vi "GetSelectedRelayCycles.vi"(2 "error in (no error)":errorcluster) -> (0 "error out":errorcluster, 1 "StringOfRelayCycles":string)   [LabVIEW 2009]
doc: "Produce a string containing about 15 cycle counts from selected relays"
panel:
  out "AT3_10dB7141RelayCycles 2":i32
  out "S2ToTransferSw5141RelayCycles":i32
  out "S1ToTransferSw5166RelayCycles":i32
  out "TxDetector1038RelayCycles":i32
  out "TxDisable7221RelayCycles":i32
  out "WGOutToAnt7206RelayCycles":i32
  out "Pwr15Supply1039RelayCycles":i32
  out "BoxInTemp1019RelayCycles":i32
  out "TransferSw7121RelayCycles":i32
  out "AT5_2dBSteps7161RelayCycles":i32
  out "AT4_10dBSteps7165RelayCycles":i32
  out "AmpBypass7201RelayCycles":i32
  out "S3toSpllitter5123RelayCycles":i32
  out "S5toPwrSensor7103RelayCycles":i32
  out "S4toSigGen5102RelayCycles":i32
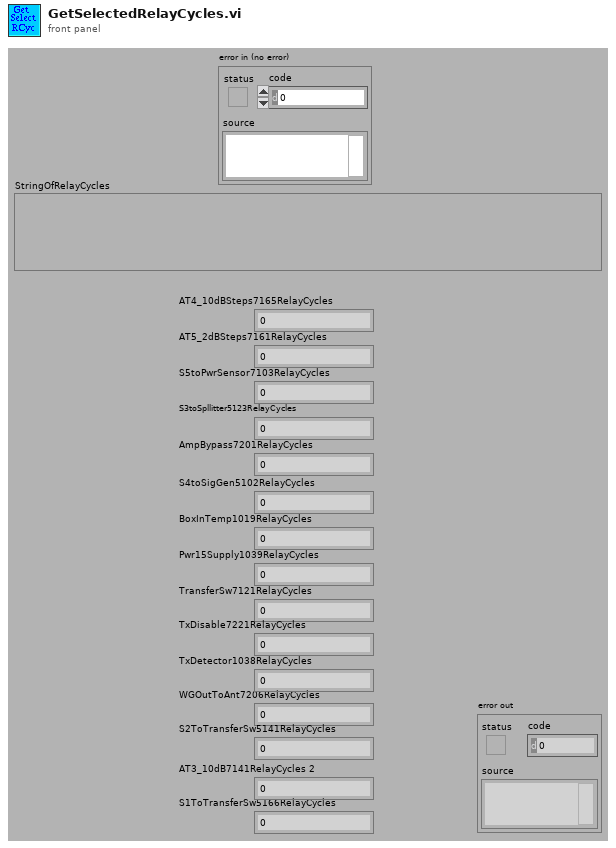
[diagram p1: front panel]
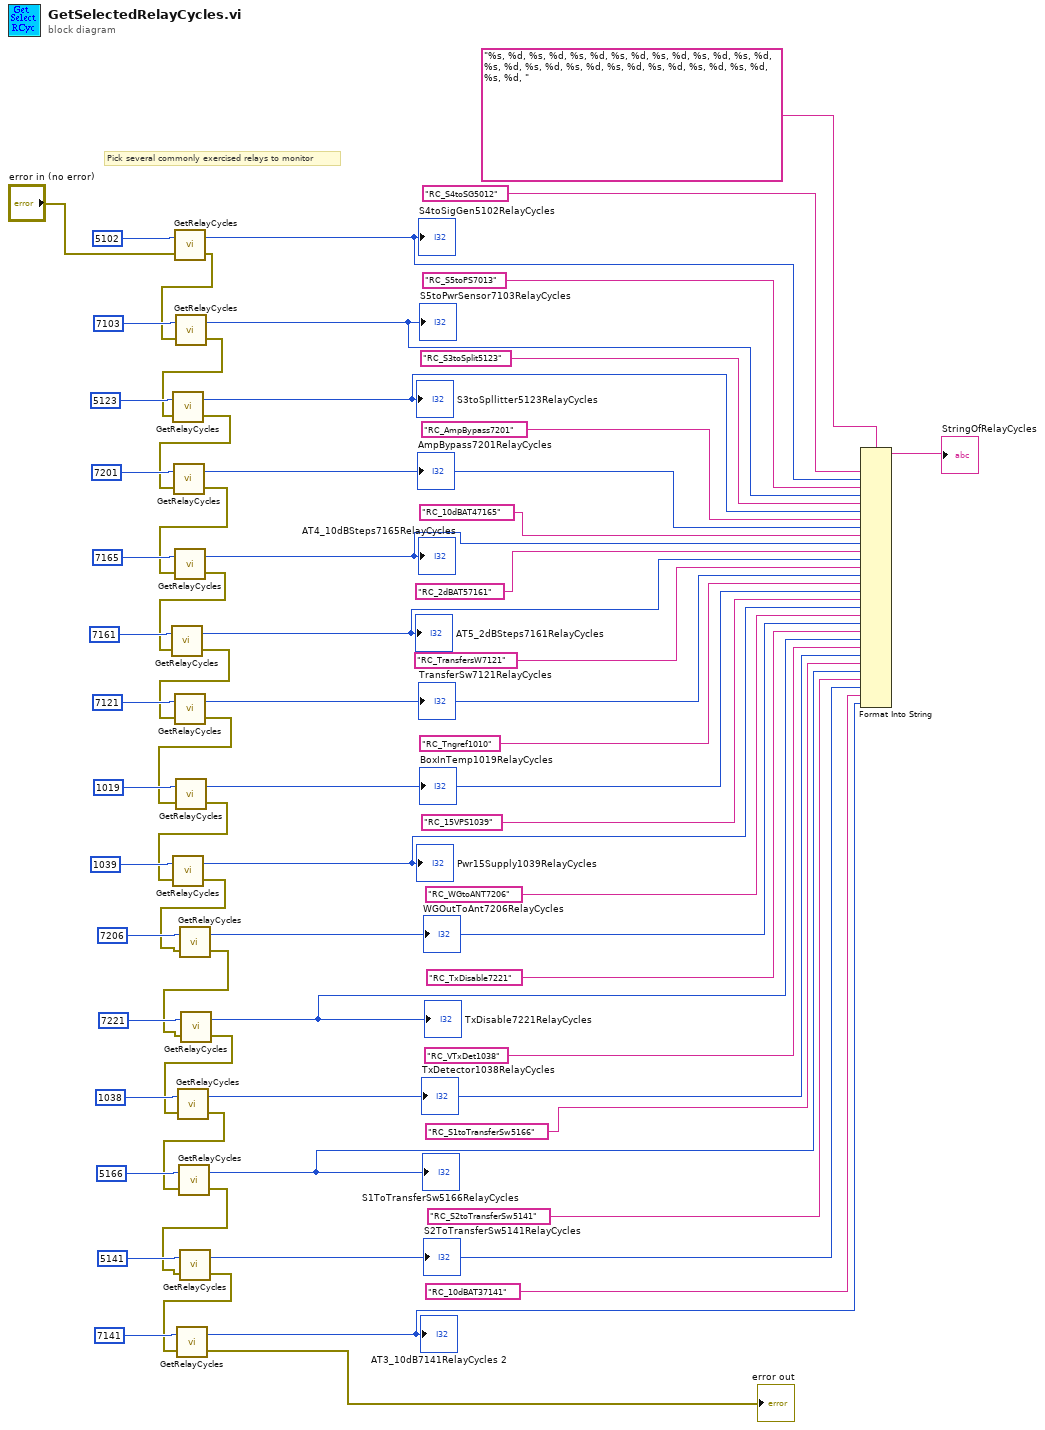
[diagram p0: block diagram]
diagram:
  # "Pick several commonly exercised relays to monitor"
  n1 = call "GetRelayCycles.vi"("error in (no error)"="error in (no error)", "Channel ID"=5102) -> ("error out"=w50:errorcluster, "N cycles"=w29:i32)
  "S4toSigGen5102RelayCycles" <- w29
  n2 = call "GetRelayCycles.vi"("error in (no error)"=w50, "Channel ID"=7103) -> ("error out"=w49:errorcluster, "N cycles"=w28:i32)
  "S5toPwrSensor7103RelayCycles" <- w28
  n3 = call "GetRelayCycles.vi"("error in (no error)"=w49, "Channel ID"=5123) -> ("error out"=w48:errorcluster, "N cycles"=w25:i32)
  "S3toSpllitter5123RelayCycles" <- w25
  n4 = call "GetRelayCycles.vi"("error in (no error)"=w48, "Channel ID"=7201) -> ("error out"=w47:errorcluster, "N cycles"=w23:i32)
  "AmpBypass7201RelayCycles" <- w23
  n5 = call "GetRelayCycles.vi"("error in (no error)"=w47, "Channel ID"=7165) -> ("error out"=w46:errorcluster, "N cycles"=w22:i32)
  "AT4_10dBSteps7165RelayCycles" <- w22
  n6 = call "GetRelayCycles.vi"("error in (no error)"=w46, "Channel ID"=7161) -> ("error out"=w45:errorcluster, "N cycles"=w19:i32)
  "AT5_2dBSteps7161RelayCycles" <- w19
  n7 = call "GetRelayCycles.vi"("error in (no error)"=w45, "Channel ID"=7121) -> ("error out"=w44:errorcluster, "N cycles"=w17:i32)
  "TransferSw7121RelayCycles" <- w17
  n8 = call "GetRelayCycles.vi"("error in (no error)"=w44, "Channel ID"=1019) -> ("error out"=w43:errorcluster, "N cycles"=w16:i32)
  "BoxInTemp1019RelayCycles" <- w16
  n9 = call "GetRelayCycles.vi"("error in (no error)"=w43, "Channel ID"=1039) -> ("error out"=w42:errorcluster, "N cycles"=w13:i32)
  "Pwr15Supply1039RelayCycles" <- w13
  n10 = call "GetRelayCycles.vi"("error in (no error)"=w42, "Channel ID"=7206) -> ("error out"=w41:errorcluster, "N cycles"=w11:i32)
  "WGOutToAnt7206RelayCycles" <- w11
  n11 = call "GetRelayCycles.vi"("error in (no error)"=w41, "Channel ID"=7221) -> ("error out"=w40:errorcluster, "N cycles"=w9:i32)
  "TxDisable7221RelayCycles" <- w9
  n12 = call "GetRelayCycles.vi"("error in (no error)"=w40, "Channel ID"=1038) -> ("error out"=w32:errorcluster, "N cycles"=w7:i32)
  "TxDetector1038RelayCycles" <- w7
  n13 = call "GetRelayCycles.vi"("error in (no error)"=w32, "Channel ID"=5166) -> ("error out"=w35:errorcluster, "N cycles"=w5:i32)
  "S1ToTransferSw5166RelayCycles" <- w5
  n14 = call "GetRelayCycles.vi"("error in (no error)"=w35, "Channel ID"=5141) -> ("error out"=w34:errorcluster, "N cycles"=w3:i32)
  "S2ToTransferSw5141RelayCycles" <- w3
  n15 = call "GetRelayCycles.vi"("error in (no error)"=w34, "Channel ID"=7141) -> ("error out"=→"error out":errorcluster, "N cycles"=w1:i32)
  "AT3_10dB7141RelayCycles 2" <- w1
  n16 = Format Into String(format string="%s, %d, %s, %d, %s, %d, %s, %d, %s, %d, %s, %d, %s, %d, %s, %d, %s, %d, %s, %d, %s, %d, %s, %d, %s, %d, %s, %d, %s, %d, ", "RC_S4toSG5012", w29, "RC_S5toPS7013", w28, "RC_S3toSplit5123", w25, "RC_AmpBypass7201", w23, "RC_10dBAT47165", w22, "RC_2dBAT57161", w19, "RC_TransfersW7121", w17, "RC_Tngref1010", w16, "RC_15VPS1039", w13, "RC_WGtoANT7206", w11, "RC_TxDisable7221", w9, "RC_VTxDet1038", w7, "RC_S1toTransferSw5166", w5, "RC_S2toTransferSw5141", w3, "RC_10dBAT37141", w1) -> (resulting string=→"StringOfRelayCycles":string)  [unwired: 2 in, 1 out]
